vi "Queue_WaitForEnqueue.vi"(8 "error in (no error)":errorcluster, 10 "Queue in":refnum<queue>, 11 "HttpResponseMessage in":refnum<class "HttpResponseMessage.lvclass">) -> (0 "error out":errorcluster)   [LabVIEW 2018, in "HttpClient_NET.lvlib" / "HttpClient_NET.lvclass"]
doc: "<b> </b> <b> </b>\nHttpClient_NET\nJustin Young - Viviota\nCopyright (c) 2021\nLicense: BSD"
uses:
  HttpClient_NET.lvclass
  HttpResponseMessage/Types/ResponseMessage_Cluster.ctl
  HttpResponseMessage/HttpResponseMessage.lvclass
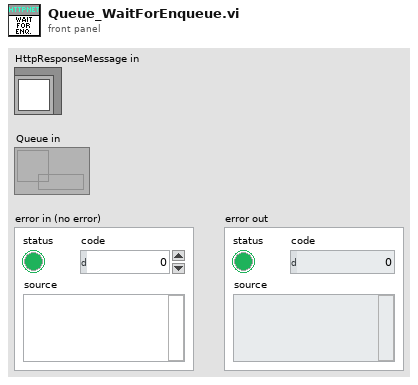
[diagram p1: front panel]
types:
  T1 = cluster{"HttpResponseMessage out":refnum<class "HttpResponseMessage.lvclass">, bool}
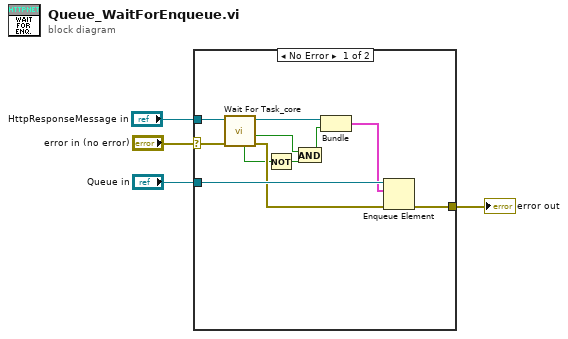
[diagram p0: block diagram]
diagram:
  n1 = case shown="No Error" "error in (no error)" {
    selector: "error in (no error)" -> [w7 w16]
    tunnel: [w15 w16] -> w4
    tunnel: "Queue in" -> [w14 _]
    tunnel: "HttpResponseMessage in" -> [w11 _]
    frame No Error {
      n2 = call "Wait For Task_core.vi"("error in (no error)"=w7, "HttpResponseMessage in"=w11) -> ("error out"=w8:errorcluster, "IsCompleted"=w9:bool, "HttpResponseMessage out"=w10:refnum<class "HttpResponseMessage.lvclass">, "Timeout"=w6:bool)  [unwired: 6 in]
      n3 = Not(x=w6) -> (.not. x?=w12:bool)
      n4 = And(x=w9, y=w12) -> (x .and. y?=w13:bool)
      n5 = Bundle("HttpResponseMessage out"=w10, w13) -> (w5:T1)  [unwired: 1 in]
      n6 = Enqueue Element(queue=w14, element=w5, error in (no error)=w8) -> (error out=w15:errorcluster)  [unwired: 1 in, 2 out]
    }
    frame Error {
    }
  }
  "error out" <- w4
